vi "recordChannels.vi"(0 "Save":bool, 1 "triggerStart":bool, 2 "TDMS File Path":path=path "E:/Sabrina/data/debug/debug", 3 "Display":bool=TRUE) -> ()   [LabVIEW 2014, in "userLibraryCustomized.lvlib"]
uses:
  userLibraryCustomized.lvlib
  <vilib>/Utility/error.llb/DialogType.ctl
  Global_stopRecordChannel.vi
  <vilib>/DAQmx/create/channels.llb/DAQmx Create Channel (AI-Voltage-Basic).vi
  <vilib>/DAQmx/configure/timing.llb/DAQmx Timing (Sample Clock).vi
  <vilib>/DAQmx/configure/task.llb/DAQmx Configure Logging (TDMS).vi
  <vilib>/DAQmx/configure/trigger.llb/DAQmx Start Trigger (Digital Edge).vi
  <vilib>/DAQmx/configure/trigger.llb/DAQmx Start Trigger (Analog Edge).vi
  <vilib>/DAQmx/create/channels.llb/DAQmx Create Channel (CI-Position-Angular Encoder).vi
  <vilib>/DAQmx/read.llb/DAQmx Read (Analog 2D DBL NChan NSamp).vi
  <vilib>/DAQmx/read.llb/DAQmx Read (Counter 1D DBL 1Chan NSamp).vi
  Global_stopExternalClock.vi
  <resource>/objmgr/daqmx.rc
panel:
  out "TDMS File Path 1":path=path "E:/Sabrina/data/debug_voltage/debug_counter.tdms"
  out "TDMS File Path 2":path=path "E:/Sabrina/data/debug_voltage/debug_counter.tdms"
  in  "Tab Control":T1(tab)
  out "Logging Mode":i32(ring)=10231 items=["Off"=10231, "Log and Read"=15842]
  in  "Speed bin (sec)":dbl=0.1
  in  "Display length (sec)":i32=6
  in  "# of Channel":i32=3
  out "Waveform Graph":dbl[][](graph)
  in  "Samples per loop":i32=1000
  in  "Sample Rate":dbl=1000.0
  in  "Sample Clock Source":tag="/Dev1/Ctr3InternalOutput"
  out "Actual Analog Sample Rate":dbl=1000.0 format="%0.2f"
  in  "Timeout (sec)":dbl=60.0 format="%#_13g"
  in  "Stop":bool
  in  "Terminal Configuration":i32(ring)=10083 items=["default"=-1, "RSE"=10083, "NRSE"=10078, "Differential"=10106, "Pseudodifferential"=12529]
  in  "Max Voltage":dbl=5.0
  in  "Min Voltage":dbl=-5.0
  in  "Physical Channel":tag="Dev1/ai0:2"
  in  "Trigger Type 2":T2(tab)
  in  "Edge 2":i32(ring)=10280 items=["Rising"=10280, "Falling"=10171]
  in  "Digital Trigger Source 2":tag="/Dev1/PFI12"
  in  "Level (V)":dbl format="%0.2f"
  in  "Hysteresis (V)":dbl
  in  "Slope":i32(ring)=10280 items=["Rising"=10280, "Falling"=10171]
  in  "Analog Trigger Source":string="APFI0"
  in  "decoding type":i32(ring)=10092 items=["X1"=10090, "X2"=10091, "X4"=10092, "Two Pulse Counting"=10313]
  in  "Z Index Terminal":tag="/Dev1/PFI7"
  in  "Z Index Enable":bool
  in  "Pulses Per Revolution":u32=360
  in  "B Input Terminal":tag="/Dev1/PFI9"
  in  "A Input Terminal":tag="PFI8"
  in  "counter":tag="Dev1/ctr1"
  in  "Trigger Type 3":enum32{"No Trigger", "Digital Arm Start"}(tab)
  in  "Edge 3":i32(ring)=10280 items=["Rising"=10280, "Falling"=10171]
  in  "Digital Trigger Source 3":tag="/Dev1/PFI2"
  in  "Trigger Type":T3(tab)
  in  "Edge":i32(ring)=10280 items=["Rising"=10280, "Falling"=10171]
  in  "Digital Trigger Source":tag="/Dev1/PFI14"
  in  "Pause When":i32(ring)=10192 items=["High"=10192, "Low"=10214]
  in  "Pause Trigger Source":tag
  out "Actual Frequency":dbl
  in  "Frequency":dbl=1000.0 format="%.6f"
  in  "counter_clock":tag="Dev1/ctr3"
  # "Timing Settings"
  # "Logging Settings"
  # "Channel Settings"
  # "Trigger Settings"
  # "To configure and use a start trigger you must have the necessary tab selected above.  Not all hardware supports triggering--refer to your device documentation for more info."
  # "Channel Settings"
  # "Trigger Settings"
  # "To configure and use a trigger or the count reset you must have the necessary tab selected above.  Not all hardware supports the above options--refer to your device documentation for more info."
  # "Trigger Settings"
  # "To configure and use a trigger you must have the necessary tab selected above."
  # "To configure and use a trigger you must have the necessary tab selected above."
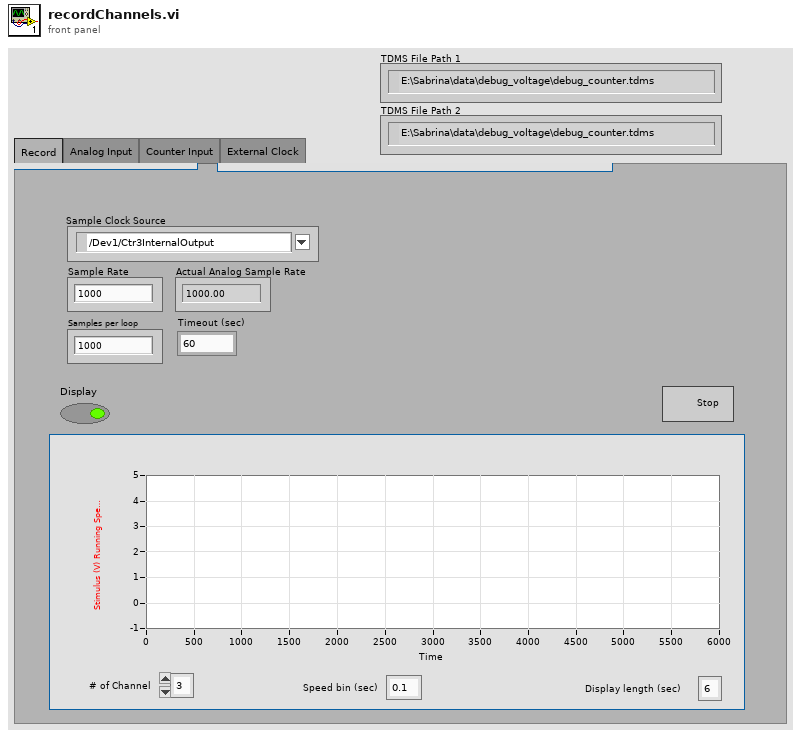
[diagram p1: front panel]
types:
  T1 = enum32{"Record", "Analog Input", "Counter Input", "External Clock"}
  T2 = enum32{"No Trigger", "Digital Start", "Analog Start"}
  T3 = enum32{"No Trigger", "Digital Start", "Digital Pause"}
  T4 = typedef "DialogType.ctl" = u16
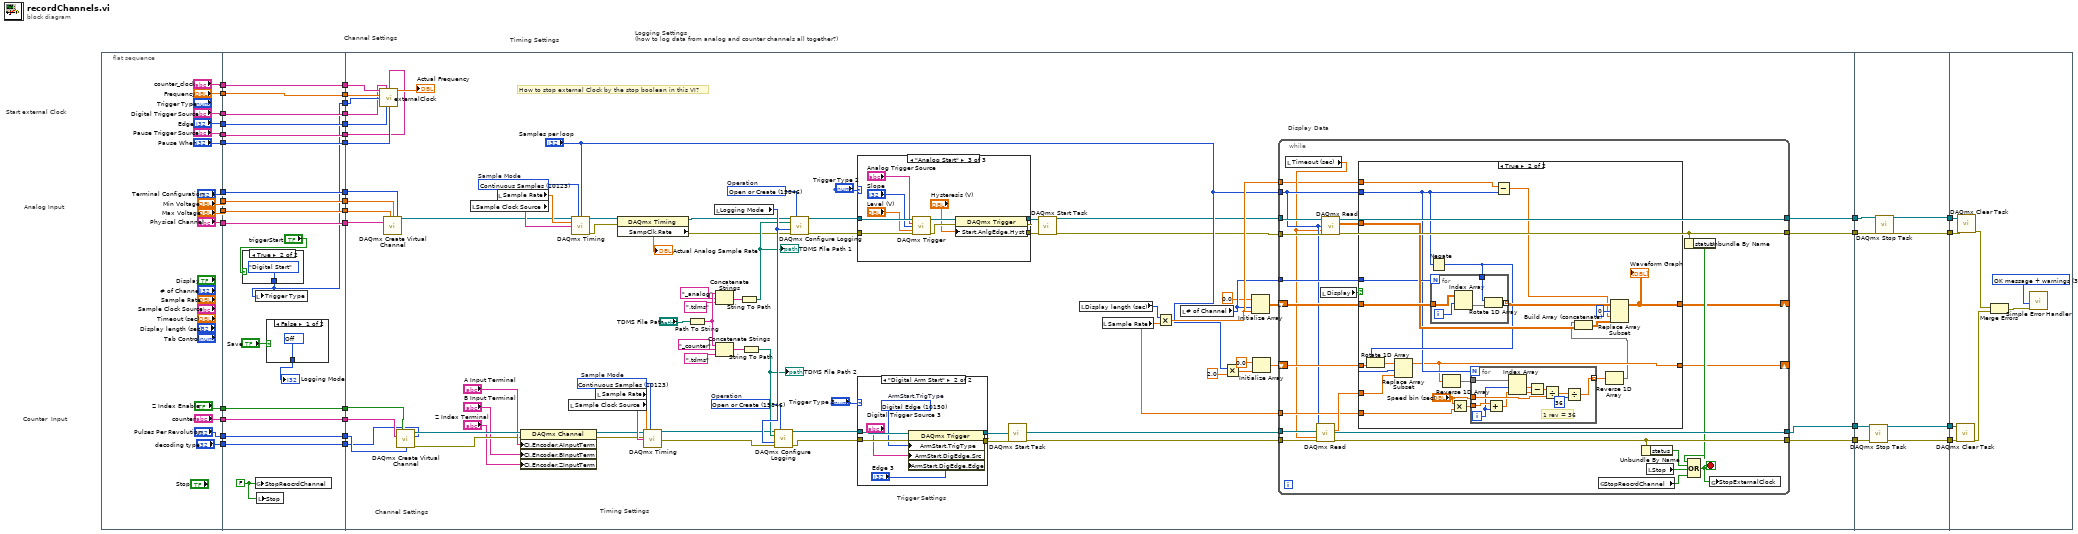
[diagram p0: block diagram]
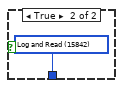
[diagram p2: hidden frame]
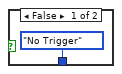
[diagram p3: hidden frame]
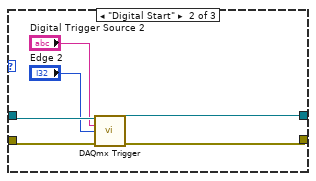
[diagram p7: hidden frame]
diagram:
  # "Timing Settings"
  # "Channel Settings"
  # "Logging Settings\n(how to log data from analog and counter channels all together?)"
  # "Start external Clock"
  # "Counter  Input"
  # "Analog Input"
  n1 = flat-sequence {
    tunnel: ["Pulses Per Revolution"] -> w37
    tunnel: ["Z Index Enable"] -> w36
    tunnel: ["counter"] -> w35
    tunnel: ["Terminal Configuration"] -> w34
    tunnel: ["Min Voltage"] -> w33
    tunnel: ["Max Voltage"] -> w32
    tunnel: ["Physical Channel"] -> w31
    tunnel: ["counter_clock"] -> w30
    tunnel: ["Frequency"] -> w29
    tunnel: ["Digital Trigger Source"] -> w28
    tunnel: ["Edge"] -> w27
    tunnel: ["Pause Trigger Source"] -> w26
    tunnel: ["Pause When"] -> w25
    tunnel: ["decoding type"] -> w1
    tunnel: w37 -> [w70]
    tunnel: w36 -> [w69]
    tunnel: w35 -> [w68]
    tunnel: w34 -> [w67]
    tunnel: w33 -> [w66]
    tunnel: w32 -> [w65]
    tunnel: w31 -> [w64]
    tunnel: w30 -> [w63]
    tunnel: w29 -> [w62]
    tunnel: w28 -> [w57]
    tunnel: w27 -> [w61]
    tunnel: w26 -> [w60]
    tunnel: w25 -> [w59]
    tunnel: [w70] -> w24
    tunnel: [w69] -> w23
    tunnel: [w68] -> w22
    tunnel: [w67] -> w21
    tunnel: [w66] -> w20
    tunnel: [w65] -> w19
    tunnel: [w64] -> w18
    tunnel: [w63] -> w17
    tunnel: [w62] -> w16
    tunnel: [w61] -> w15
    tunnel: [w60] -> w14
    tunnel: [w59] -> w13
    tunnel: [w53] -> w12
    tunnel: [w57] -> w11
    tunnel: [w52] -> w2
    tunnel: w1 -> [w52]
    tunnel: w24 -> [w80]
    tunnel: w23 -> [w82]
    tunnel: w22 -> [w81]
    tunnel: w21 -> [w86]
    tunnel: w20 -> [w85]
    tunnel: w19 -> [w84]
    tunnel: w18 -> [w83]
    tunnel: w17 -> [w93]
    tunnel: w16 -> [w89]
    tunnel: w15 -> [w90]
    tunnel: w14 -> [w91]
    tunnel: w13 -> [w92]
    tunnel: w12 -> [w88]
    tunnel: w11 -> [w87]
    tunnel: [w78] -> w10
    tunnel: [w76] -> w8
    tunnel: [w77] -> w7
    tunnel: [w79] -> w6
    tunnel: w2 -> [w75]
    tunnel: w10 -> [w249]
    tunnel: [w250] -> w9
    tunnel: w8 -> [w250]
    tunnel: w7 -> [w248]
    tunnel: w6 -> [w247]
    tunnel: [w249] -> w5
    tunnel: [w246] -> w4
    tunnel: [w245] -> w3
    tunnel: w9 -> [w253]
    tunnel: w5 -> [w256]
    tunnel: w4 -> [w255]
    tunnel: w3 -> [w254]
    frame #0 {
    }
    frame #1 {
      w54 = FALSE
      n2 = case shown="True" "triggerStart" {
        tunnel: [T3."No Trigger" ("Trigger Type") T3."Digital Start" ("Trigger Type")] -> w53
        frame False {
        }
        frame True {
        }
      }
      n3 = local write "Trigger Type"(w53) -> ()
      n4 = global write "Global_stopRecordChannel.vi" "StopReocrdChannel"(w54) -> ()
      n5 = local write "Stop"(w54) -> ()
      n6 = case shown="False" "Save" {
        tunnel: [w71 w72] -> w56
        frame False {
          w71 = 10231 items=["Off"=10231, "Log and Read"=15842] ("Logging Mode")
        }
        frame True {
          w72 = 15842 items=["Off"=10231, "Log and Read"=15842] ("Logging Mode")
        }
      }
      "Logging Mode" <- w56
    }
    frame #2 {
      w128 = 15846 items=["Open"=10437, "Open or Create"=15846, "Create or Replace"=15847, "Create"=15848]  # Operation
      w127 = 15846 items=["Open"=10437, "Open or Create"=15846, "Create or Replace"=15847, "Create"=15848]  # Operation
      w120 = 10123 items=["Finite Samples"=10178, "Continuous Samples"=10123, "Hardware Timed Single Point"=12522]  # Sample Mode
      w103 = 10123 items=["Finite Samples"=10178, "Continuous Samples"=10123, "Hardware Timed Single Point"=12522]  # Sample Mode
      # "Channel Settings"
      # "Display Data"
      # "How to stop external Clock by the stop boolean in this VI?"
      # "Trigger Settings"
      # "Timing Settings"
      n7 = call "externalClock.vi"("Counter"=w93, "Digital Trigger Source"=w87, "Pause Trigger Source"=w91, "Frequency"=w89, "Trigger Type"=w88, "Edge"=w90, "Pause When"=w92) -> ("Actual Frequency"=→"Actual Frequency":dbl)  [unwired: 8 in]
      n8 = call-poly <vilib>:"DAQmx Create Virtual Channel.vi"("maximum value"=w84, "minimum value"=w85, "input terminal configuration"=w86, "physical channels"=w83) -> ("task out"=w94:refnum<k21>)  [unwired: 10 in, 1 out]
      n9 = call-poly <vilib>:"DAQmx Create Virtual Channel.vi"("z index enable"=w82, "counter"=w81, "decoding type"=w75, "pulses per revolution"=w80) -> ("task out"=w114:refnum<k21>, "error out"=w112:errorcluster)  [unwired: 10 in]
      n10 = local read "Sample Clock Source"() -> (w107:tag)
      n11 = local read "Sample Rate"() -> (w106:dbl)
      n12 = property class="DAQmx Channel"(reference=w114, error in=w112, "CI.Encoder.AInputTerm"="A Input Terminal", "CI.Encoder.BInputTerm"="B Input Terminal", "CI.Encoder.ZInputTerm"="Z Index Terminal") -> (reference out=w110:refnum<k21>, error out=w109:errorcluster)
      n13 = local read "Sample Clock Source"() -> (w122:tag)
      n14 = call-poly <vilib>:"DAQmx Timing.vi"("task/channels in"=w94, "sample mode"=w103, "samples per channel"="Samples per loop", "rate"=w106, "source"=w107) -> ("task out"=w105:refnum<k21>, "error out"=w104:errorcluster)  [unwired: 9 in]
      n15 = local read "Sample Rate"() -> (w121:dbl)
      n16 = property class="DAQmx Timing"(reference=w105, error in=w104) -> (reference out=w102:refnum<k21>, error out=w101:errorcluster, "SampClk.Rate"=→"Actual Analog Sample Rate":dbl)
      n17 = call-poly <vilib>:"DAQmx Timing.vi"("task/channels in"=w110, "sample mode"=w120, "rate"=w121, "source"=w122, "error in"=w109) -> ("task out"=w131:refnum<k21>, "error out"=w129:errorcluster)  [unwired: 9 in]
      n18 = Path To String(path="TDMS File Path") -> (string=w151:string)
      n19 = local read "Logging Mode"() -> (w153:i32)
      n20 = Concatenate Strings(w151, "_analog" ("string"), ".tdms" ("regular expression (\"\")")) -> (w147:string)
      n21 = Concatenate Strings(w151, "_counter" ("string"), ".tdms" ("regular expression (\"\")")) -> (w148:string)
      n22 = String To Path(string=w147) -> (path=w149:path)
      "TDMS File Path 1" <- w149
      n23 = String To Path(string=w148) -> (path=w150:path)
      "TDMS File Path 2" <- w150
      n24 = call-poly <vilib>:"DAQmx Configure Logging.vi"("task/channels in"=w131, "operation"=w128, "file path"=w150, "logging mode"=w153, "error in"=w129) -> ("task out"=w132:refnum<k21>, "error out"=w130:errorcluster)  [unwired: 9 in]
      n25 = call-poly <vilib>:"DAQmx Configure Logging.vi"("task/channels in"=w102, "operation"=w127, "file path"=w149, "logging mode"=w153, "error in"=w101) -> ("task out"=w100:refnum<k21>, "error out"=w99:errorcluster)  [unwired: 9 in]
      n26 = case shown="\"Analog Start\"" "Trigger Type 2" {
        tunnel: w100 -> [w228 w234 w244]
        tunnel: w99 -> [w227 w233 w243]
        tunnel: [w228 w232 w241] -> w98
        tunnel: [w227 w231 w240] -> w97
        frame "No Trigger", Default {
        }
        frame "Digital Start" {
          n27 = call-poly <vilib>:"DAQmx Trigger.vi"("task/channels in"=w234, "source"="Digital Trigger Source 2", "edge"="Edge 2", "error in"=w233) -> ("task out"=w232:refnum<k21>, "error out"=w231:errorcluster)  [unwired: 10 in]
        }
        frame "Analog Start" {
          n28 = call-poly <vilib>:"DAQmx Trigger.vi"("task/channels in"=w244, "source"="Analog Trigger Source", "slope"="Slope", "level"="Level (V)", "error in"=w243) -> ("task out"=w239:refnum<k21>, "error out"=w238:errorcluster)  [unwired: 9 in]
          n29 = property class="DAQmx Trigger"(reference=w239, error in=w238, "Start.AnlgEdge.Hyst"="Hysteresis (V)") -> (reference out=w241:refnum<k21>, error out=w240:errorcluster)
        }
      }
      n30 = case shown="\"Digital Arm Start\"" "Trigger Type 3" {
        tunnel: w132 -> [w219 w226]
        tunnel: w130 -> [w218 w223]
        tunnel: [w219 w225] -> w115
        tunnel: [w218 w224] -> w116
        frame "No Trigger", Default {
        }
        frame "Digital Arm Start" {
          w220 = 10150 items=["Digital Edge"=10150, "None"=10230]  # ArmStart.TrigType
          n31 = property class="DAQmx Trigger"(reference=w226, error in=w223, "ArmStart.TrigType"=w220, "ArmStart.DigEdge.Src"="Digital Trigger Source 3", "ArmStart.DigEdge.Edge"="Edge 3") -> (reference out=w225:refnum<k21>, error out=w224:errorcluster)
        }
      }
      n32 = call <vilib>:"DAQmx Start Task.vi"("task/channels in"=w115, "error in"=w116) -> ("task out"=w119:refnum<k21>, "error out"=w118:errorcluster)  [unwired: 12 in]
      n33 = call <vilib>:"DAQmx Start Task.vi"("task/channels in"=w98, "error in"=w97) -> ("task out"=w123:refnum<k21>, "error out"=w124:errorcluster)  [unwired: 12 in]
      n34 = local read "Display length (sec)"() -> (w152:i32)
      n35 = local read "Sample Rate"() -> (w140:dbl)
      n36 = Multiply(x=w152, y=w140) -> (x*y=w141:dbl)
      n37 = local read "# of Channel"() -> (w135:i32)
      n38 = Multiply(x="Samples per loop", y=2.0) -> (x*y=w137:dbl)
      n39 = Initialize Array(0.0 ("element"), w135, w141) -> (w134:dbl[][])
      n40 = Initialize Array(0.0 ("element"), w137) -> (w139:dbl[])
      n41 = while {
        tunnel: w119 -> [w178]
        tunnel: w118 -> [w177]
        tunnel: [w175] -> w76
        tunnel: [w176] -> w77
        tunnel: w123 -> [w173]
        tunnel: w124 -> [w174]
        tunnel: "Samples per loop" -> [w161]
        tunnel: [w172] -> w79
        tunnel: [w171] -> w78
        shift-right: [w166] -> _
        shift-left: w134 -> [w168]
        tunnel: w135 -> [w165]
        tunnel: w141 -> [w158]
        shift-right: [w159] -> _
        shift-left: w139 -> [w164]
        tunnel: w140 -> [w162]
        stop <- w154 stop-if-true
        n42 = local read "Timeout (sec)"() -> (w160:dbl)
        n43 = call-poly <vilib>:"DAQmx Read.vi"("task/channels in"=w178, "number of samples per channel"=w161, "timeout"=w160, "error in"=w177) -> ("task out"=w176:refnum<k21>, "data"=w163:dbl[], "error out"=w175:errorcluster)  [unwired: 9 in]
        n44 = local read "Display"() -> (w157:bool)
        n45 = call-poly <vilib>:"DAQmx Read.vi"("task/channels in"=w173, "number of samples per channel"=w161, "timeout"=w160, "error in"=w174) -> ("task out"=w172:refnum<k21>, "data"=w167:dbl[][], "error out"=w171:errorcluster)  [unwired: 9 in]
        n46 = case shown="True" w157 {
          tunnel: w168 -> [w179 w201]
          tunnel: w167 -> [_ w199]
          tunnel: [w179 w196] -> w166
          tunnel: w165 -> [_ w195]
          tunnel: w164 -> [w180 w194]
          tunnel: w163 -> [_ w192]
          tunnel: w162 -> [_ w190]
          tunnel: w161 -> [_ w186]
          tunnel: [w180 w185] -> w159
          tunnel: w158 -> [_ w183]
          frame False {
          }
          frame True {
            n47 = Negate(x=w186) -> (-x=w187:i32)
            n48 = Rotate 1D Array(1:w194, 2:w187) -> (0:w193:dbl[])
            n49 = Replace Array Subset(array=w193, new element=w192, index=w186) -> (w185:dbl[])
            n50 = for {
              N: w195 -> [_]
              tunnel: w201 -> [w216]
              tunnel: [w215] -> w200 mode=indexing
              tunnel: w187 -> [w213]
              i -> [w214]
              n51 = Index Array(array=w216, index (row)=w214) -> (element=w217:dbl[])  [unwired: 1 in]
              n52 = Rotate 1D Array(1:w217, 2:w213) -> (0:w215:dbl[])
            }
            n53 = Reverse 1D Array(array=w185) -> (reversed array=w191:dbl[])
            n54 = Multiply(x="Speed bin (sec)", y=w190) -> (x*y=w189:dbl)
            n55 = for {
              N: w186 -> [_]
              tunnel: w191 -> [w212]
              tunnel: w189 -> [w209]
              tunnel: "Speed bin (sec)" -> [w211]
              tunnel: [w202] -> w188 mode=indexing
              i -> [w208]
              # "1 rev = 36"
              n56 = Add(x=w209, y=w208) -> (x+y=w210:dbl)
              n57 = Index Array(array=w212, index #1=w208, index #2=w210) -> (element #1=w206:dbl, element #2=w207:dbl)
              n58 = Subtract(x=w206, y=w207) -> (x-y=w205:dbl)
              n59 = Divide(x=w205, y=w211) -> (x/y=w204:dbl)
              n60 = Divide(x=w204, y=36) -> (x/y=w202:dbl)
            }
            n61 = Subtract(x=w183, y=w186) -> (x-y=w184:dbl)
            n62 = Reverse 1D Array(array=w188) -> (reversed array=w181:dbl[])
            n63 = Build Array (concatenate)(w181, w199) -> (w197:dbl[][])
            n64 = Replace Array Subset(array=w200, new element=w197, index (row)=0 ("disabled index (col)"), index (col)=w184) -> (w196:dbl[][])
            "Waveform Graph" <- w196
          }
        }
        n65 = global read "Global_stopRecordChannel.vi" "StopReocrdChannel"() -> (w155:bool)
        n66 = Unbundle By Name(w175) -> ("status"=w169:bool)
        n67 = local read "Stop"() -> (w156:bool)
        n68 = Unbundle By Name(w171) -> ("status"=w170:bool)
        n69 = Compound Arithmetic op=OR(w170, w169, w156, w155) -> (w154:bool)
        n70 = global write "Global_stopExternalClock.vi" "StopExternalClock"(w154) -> ()
      }
    }
    frame #3 {
      n71 = call <vilib>:"DAQmx Stop Task.vi"("task/channels in"=w248) -> ("task out"=w245:refnum<k21>)  [unwired: 13 in, 1 out]
      n72 = call <vilib>:"DAQmx Stop Task.vi"("task/channels in"=w247) -> ("task out"=w246:refnum<k21>)  [unwired: 13 in, 1 out]
    }
    frame #4 {
      w257 = T4 3 items=["no dialog", "OK message", "continue or stop message", "OK message + warnings", "continue/stop + warnings"] ("type of dialog (OK msg:1)")
      n73 = call <vilib>:"DAQmx Clear Task.vi"("task in"=w254, "error in"=w253) -> ("error out"=w251:errorcluster)  [unwired: 13 in]
      n74 = call <vilib>:"DAQmx Clear Task.vi"("task in"=w255, "error in"=w256) -> ("error out"=w252:errorcluster)  [unwired: 13 in]
      n75 = Merge Errors(w252, w251) -> (w258:errorcluster)
      n76 = call <vilib>:"Simple Error Handler.vi"("type of dialog (OK msg:1)"=w257, "error in (no error)"=w258) -> ()  [unwired: 3 in, 5 out]
    }
  }
